vi "UI - Initiate Connection.vi"(8 "error in (no error)":errorcluster, 10 "Controller Address":string, 11 "Message Queue":refnum<queue>) -> (0 "error out":errorcluster, 1 "Connected?":bool)   [LabVIEW 2018]
uses:
  Message Queue/Message Cluster (string).ctl
  controls/Raw Values.ctl
  controls/FPGA State.ctl
  controls/Variable References.ctl
  Globals/Global - Configuration Options.vi
  Globals/Global - UI Stream and Variable Connections.vi
  Message Queue/Message Queue.lvlib
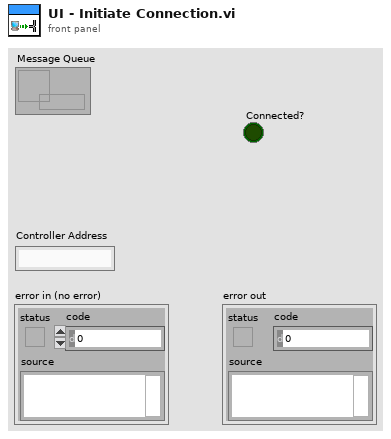
[diagram p1: front panel]
types:
  T1 = typedef "FPGA State.ctl" = enum16{"Safe State", "Control (PID)"}
  T2 = typedef "Raw Values.ctl" = cluster{"Channel 0":fxp<+/-,20,5>, "Channel 1":fxp<+/-,20,5>, "Channel 2":bool}
  T3 = typedef "Message Queue.lvlib/Message Cluster (string).ctl" = cluster{"Message":string, "Message Data":variant}
  T4 = typedef "Variable References.ctl" = cluster{"CPU Usage":refnum<k21>, "Contiguous Memory":refnum<k21>, "Input Values":refnum<k21>, "Output Values":refnum<k21>, "FPGA Mode":refnum<k21>, "Actual Loop Period":refnum<k21>}
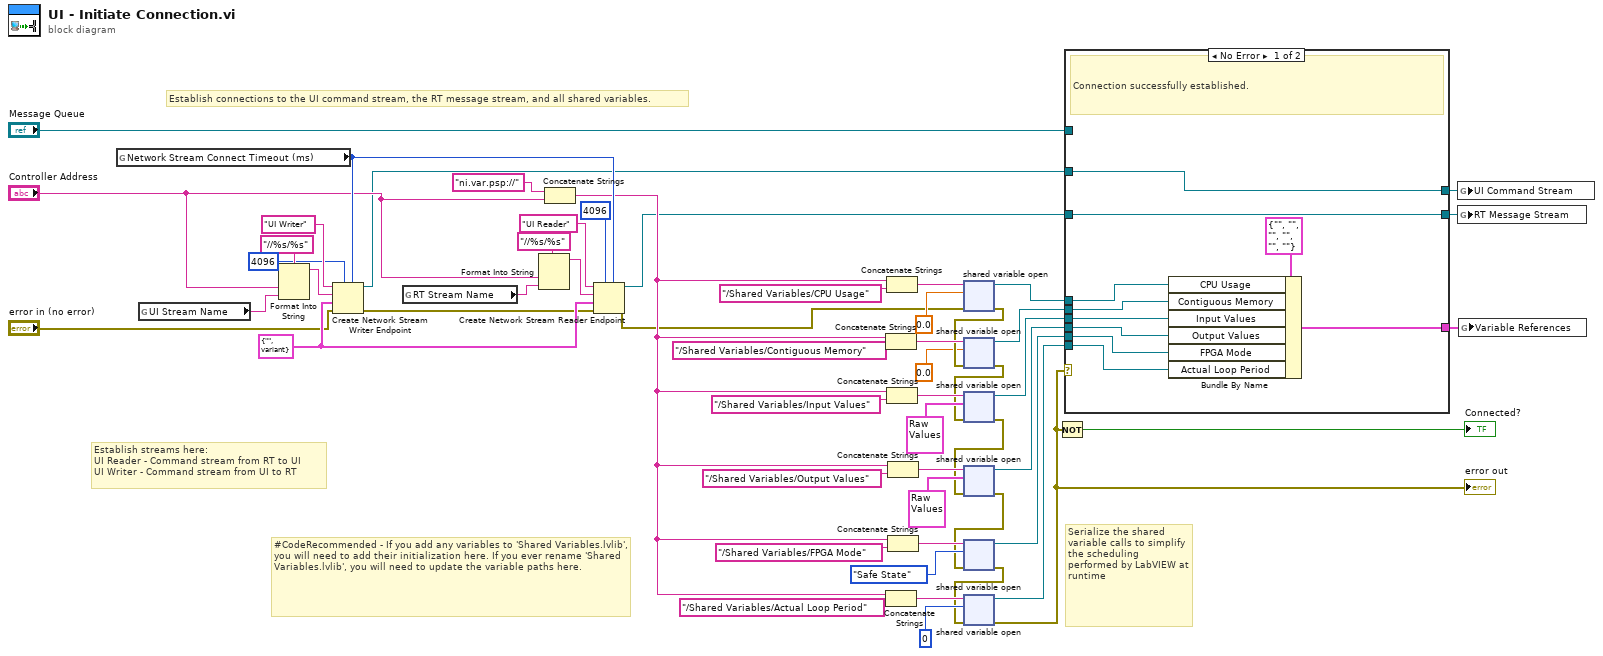
[diagram p0: block diagram]
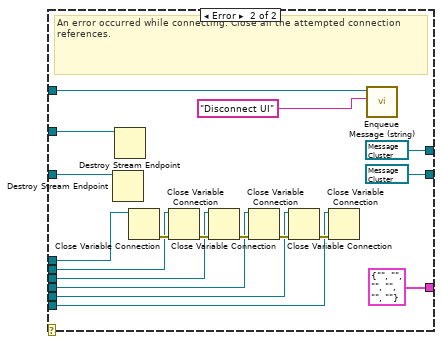
[diagram p2: hidden frame]
diagram:
  w46 = T3 {"Message"="", "Message Data"=variant} ("Message Cluster")
  # "Establish connections to the UI command stream, the RT message stream, and all shared variables."
  # "#CodeRecommended - If you add any variables to 'Shared Variables.lvlib', you will need to add their initialization here. If you ever rename 'Shared Variables.lvlib', you will need to update the variable paths here."
  # "Establish streams here:\nUI Reader - Command stream from RT to UI\nUI Writer - Command stream from UI to RT"
  # "Serialize the shared variable calls to simplify the scheduling performed by LabVIEW at runtime"
  n1 = global read "Global - Configuration Options.vi" "Network Stream Connect Timeout (ms)"() -> (w45:i32)
  n2 = global read "Global - Configuration Options.vi" "UI Stream Name"() -> (w53:string)
  n3 = Format Into String(format string="//%s/%s", "Controller Address", w53) -> (resulting string=w52:string)  [unwired: 2 in, 1 out]
  n4 = Create Network Stream Writer Endpoint(5:w45, 7:4096 ("writer buffer size"), 8:"error in (no error)", 9:w46, 10:w52, 11:"UI Writer" ("writer name")) -> (0:w6:errorcluster, 3:w12:refnum<k21>)  [unwired: 1 in]
  n5 = global read "Global - Configuration Options.vi" "RT Stream Name"() -> (w50:string)
  n6 = Format Into String(format string="//%s/%s", "Controller Address", w50) -> (resulting string=w49:string)  [unwired: 2 in, 1 out]
  n7 = Concatenate Strings("ni.var.psp://", "Controller Address") -> (w20:string)
  n8 = Create Network Stream Reader Endpoint(5:w45, 7:4096 ("reader buffer size"), 8:w6, 9:w46, 10:w49, 11:"UI Reader" ("reader name")) -> (0:w5:errorcluster, 3:w11:refnum<k21>)  [unwired: 1 in]
  n9 = Concatenate Strings(w20, "/Shared Variables/Contiguous Memory") -> (w38:string)
  n10 = Concatenate Strings(w20, "/Shared Variables/Actual Loop Period") -> (w30:string)
  n11 = Concatenate Strings(w20, "/Shared Variables/CPU Usage") -> (w41:string)
  n12 = Concatenate Strings(w20, "/Shared Variables/Input Values") -> (w36:string)
  n13 = Concatenate Strings(w20, "/Shared Variables/Output Values") -> (w34:string)
  n14 = Concatenate Strings(w20, "/Shared Variables/FPGA Mode") -> (w33:string)
  n15 = shared-variable-open(w41, w5, 0.0) -> (w18:refnum<k21>, w25:errorcluster)  [unwired: 1 in]
  n16 = shared-variable-open(w38, w25, 0.0) -> (w17:refnum<k21>, w24:errorcluster)  [unwired: 1 in]
  n17 = shared-variable-open(w36, w24, T2 {"Channel 0"=0.0, "Channel 1"=0.0, "Channel 2"=FALSE}) -> (w16:refnum<k21>, w23:errorcluster)  [unwired: 1 in]
  n18 = shared-variable-open(w34, w23, T2 {"Channel 0"=0.0, "Channel 1"=0.0, "Channel 2"=FALSE}) -> (w15:refnum<k21>, w22:errorcluster)  [unwired: 1 in]
  n19 = shared-variable-open(w33, w22, FPGA_State."Safe State" ("FPGA State")) -> (w14:refnum<k21>, w21:errorcluster)  [unwired: 1 in]
  n20 = shared-variable-open(w30, w21, u32 0) -> (w13:refnum<k21>, w19:errorcluster)  [unwired: 1 in]
  "error out" <- w19
  n21 = Not(x=w19) -> (.not. x?=→"Connected?":bool)
  n22 = case shown="No Error" w19 {
    tunnel: w18 -> [w64 w76]
    tunnel: w17 -> [w63 w71]
    tunnel: w16 -> [w62 w72]
    tunnel: w15 -> [w61 w73]
    tunnel: w14 -> [w60 w74]
    tunnel: w13 -> [w59 w75]
    tunnel: w12 -> [w56 w82]
    tunnel: w11 -> [w57 w83]
    tunnel: [w58 T4 {"CPU Usage"="", "Contiguous Memory"="", "Input Values"="", "Output Values"="", "FPGA Mode"="", "Actual Loop Period"=""} ("Variable References")] -> w10
    tunnel: [w57 refnum<k21> refnum] -> w9
    tunnel: [w56 refnum<k21> refnum] -> w8
    tunnel: "Message Queue" -> [_ w67]
    frame No Error {
      # "Connection successfully established."
      n23 = Bundle By Name(cluster=T4 {"CPU Usage"="", "Contiguous Memory"="", "Input Values"="", "Output Values"="", "FPGA Mode"="", "Actual Loop Period"=""} ("Variable References"), "CPU Usage"=w64, "Contiguous Memory"=w63, "Input Values"=w62, "Output Values"=w61, "FPGA Mode"=w60, "Actual Loop Period"=w59) -> (w58:T4)
    }
    frame Error {
      # "An error occurred while connecting. Close all the attempted connection references."
      n24 = Destroy Stream Endpoint(11:w83) -> ()  [unwired: 1 in, 1 out]
      n25 = Destroy Stream Endpoint(11:w82) -> ()  [unwired: 1 in, 1 out]
      n26 = Close Variable Connection(11:w76) -> (0:w77:errorcluster)  [unwired: 1 in]
      n27 = Close Variable Connection(8:w77, 11:w71) -> (0:w78:errorcluster)
      n28 = Close Variable Connection(8:w78, 11:w72) -> (0:w79:errorcluster)
      n29 = Close Variable Connection(8:w79, 11:w73) -> (0:w80:errorcluster)
      n30 = Close Variable Connection(8:w80, 11:w74) -> (0:w81:errorcluster)
      n31 = Close Variable Connection(8:w81, 11:w75) -> ()  [unwired: 1 out]
      n32 = call "Enqueue Message (string).vi"("Message"="Disconnect UI", "Message Queue"=w67) -> ()  [unwired: 8 in, 2 out]
    }
  }
  n33 = global write "Global - UI Stream and Variable Connections.vi" "UI Command Stream"(w8) -> ()
  n34 = global write "Global - UI Stream and Variable Connections.vi" "RT Message Stream"(w9) -> ()
  n35 = global write "Global - UI Stream and Variable Connections.vi" "Variable References"(w10) -> ()
